vi "coverage.vi"() -> ()   [LabVIEW 2020]
uses:
  <vilib>/Wiresmith Technology/G CLI/CLI Class/CLI.lvclass
panel:
  out "error out":errorcluster
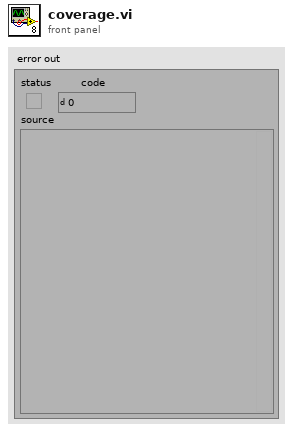
[diagram p1: front panel]
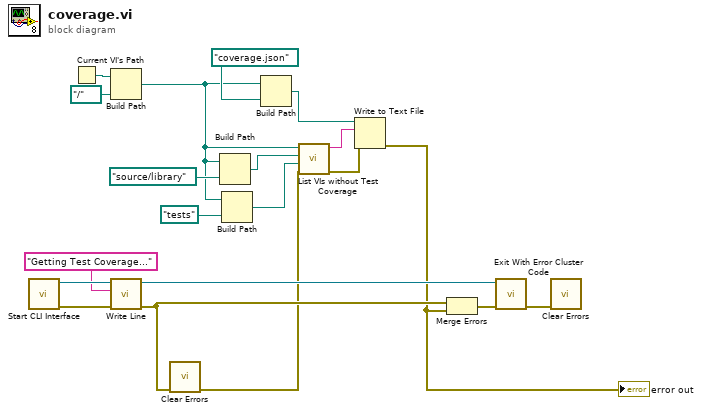
[diagram p0: block diagram]
diagram:
  n1 = call <vilib>:"Start CLI Interface.vi"() -> ("error out"=w10:errorcluster, "CLI out"=w9:refnum<class "CLI.lvclass">)  [unwired: 8 in, 2 out]
  n2 = Current VI's Path() -> (path=w16:path)
  n3 = Build Path(base path=w16, name or relative path=path "../..") -> (appended path=w1:path)
  n4 = call <vilib>:"Write Line.vi"("error in (no error)"=w10, "Text to Write"="Getting Test Coverage...", "CLI in"=w9) -> ("error out"=w5:errorcluster, "CLI out"=w7:refnum<class "CLI.lvclass">)  [unwired: 7 in]
  n5 = call <vilib>:"Clear Errors.vi"("error in (no error)"=w5) -> ("error out"=w3:errorcluster)  [unwired: 5 in, 1 out]
  n6 = Build Path(base path=w1, name or relative path=path "source/library" ("Relative path (.)")) -> (appended path=w12:path)
  n7 = Build Path(base path=w1, name or relative path=path "tests" ("Relative path (.)")) -> (appended path=w11:path)
  n8 = Build Path(base path=w1, name or relative path=path "coverage.json" ("Relative path (.)")) -> (appended path=w19:path)
  n9 = call "List VIs without Test Coverage.vi"("error in (no error)"=w3, "Tests Root"=w11, "Source Root"=w12, "Project Root"=w1) -> ("error out"=w17:errorcluster, "coverage.json"=w18:string)  [unwired: 4 in, 2 out]
  n10 = Write to Text File(file (use dialog)=w19, text=w18, error in=w17) -> (error out=w2:errorcluster)  [unwired: 1 in, 2 out]
  "error out" <- w2
  n11 = Merge Errors(w5, w2) -> (w6:errorcluster)
  n12 = call <vilib>:"Exit With Error Cluster Code.vi"("error in (no error)"=w6, "CLI in"=w7) -> ("error out"=w4:errorcluster)  [unwired: 9 in]
  n13 = call <vilib>:"Clear Errors.vi"("error in (no error)"=w4) -> ()  [unwired: 5 in, 2 out]
